vi "edittest set MN SN by PID.vi"(2 "fSpartanSetsSN":bool, 3 "FIELDS (empty)":T1[](array[typedef])) -> (1 "FIELDS out":T1[](array[typedef]))   [LabVIEW 2011]
uses:
  server/database/Fields/Field Record.ctl
  server/database/Fields/Field DataTypes.ctl
  server/database/Fields/Field NextItem.ctl
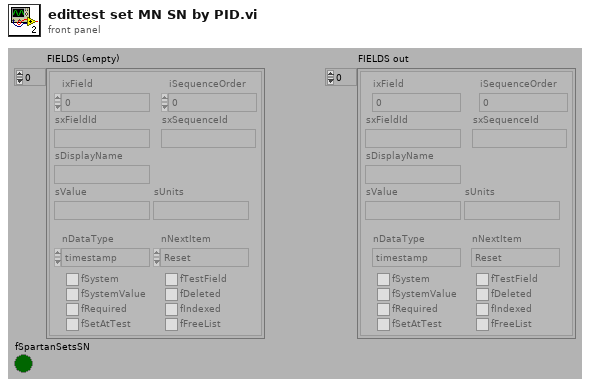
[diagram p1: front panel]
types:
  T1 = typedef "Field Record.ctl" = cluster{"ixField":i32, "iSequenceOrder":i32, "sxFieldId":string, "sxSequenceId":string, "sDisplayName":string, "sValue":string, "sUnits":string, "nDataType":T2, "nNextItem":T3, "fSystem":bool, "fSystemValue":bool, "fRequired":bool, "fSetAtTest":bool, "fTestField":bool, "fDeleted":bool, "fIndexed":bool, "fFreeList":bool}
  T2 = typedef "Field DataTypes.ctl" = enum32{"text", "numeric", "list", "timestamp", "boolean"}
  T3 = typedef "Field NextItem.ctl" = enum32{"Reset", "Retain", "Auto-Increment"}
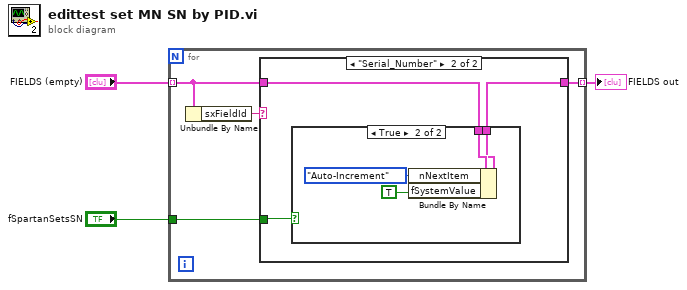
[diagram p0: block diagram]
diagram:
  n1 = for {
    tunnel: "FIELDS (empty)" -> [w6] mode=indexing
    tunnel: [w5] -> w2 mode=indexing
    tunnel: "fSpartanSetsSN" -> [w4]
    n2 = Unbundle By Name(w6) -> ("sxFieldId"=w7:string)
    n3 = case shown="\"Serial_Number\"" w7 {
      tunnel: w6 -> [w8 w11]
      tunnel: [w8 w10] -> w5
      tunnel: w4 -> [_ w9]
      frame Default {
      }
      frame "Serial_Number" {
        n4 = case shown="True" w9 {
          tunnel: w11 -> [w12 w16]
          tunnel: [w12 w15] -> w10
          frame False {
          }
          frame True {
            n5 = Bundle By Name(cluster=w16, "nNextItem"=Field_NextItem."Auto-Increment", "fSystemValue"=TRUE ("fSystem")) -> (w15:T1)
          }
        }
      }
    }
  }
  "FIELDS out" <- w2
